vi "Array.vi"() -> ()   [LabVIEW 2018]
panel:
  in  "length":i32
  in  "index":i32
  in  "Mult":dbl
  out "Sub Array":dbl[](array[numeric])
  out "Array final":dbl[](array[numeric])
  out "Array":dbl[](array[numeric])
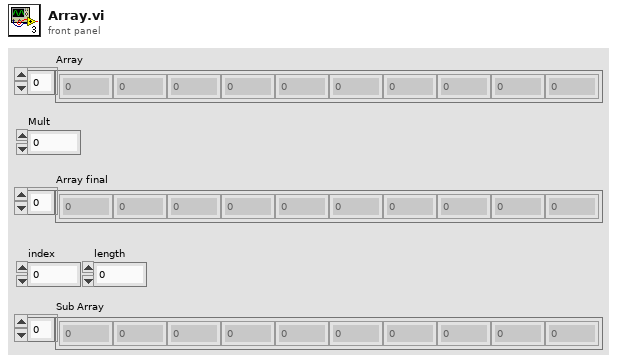
[diagram p1: front panel]
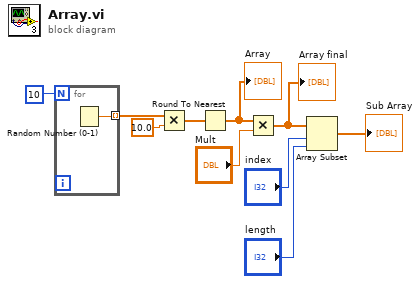
[diagram p0: block diagram]
diagram:
  n1 = for {
    N: 10 -> [_]
    tunnel: [w11] -> w1 mode=indexing
    n2 = Random Number (0-1)() -> (number: 0 to 1=w11:dbl)
  }
  n3 = Multiply(x=w1, y=10.0) -> (x*y=w3:dbl[])
  n4 = Round To Nearest(number=w3) -> (nearest integer value=w2:dbl[])
  "Array" <- w2
  n5 = Multiply(x=w2, y="Mult") -> (x*y=w8:dbl[])
  "Array final" <- w8
  n6 = Array Subset(array=w8, index="index", length="length") -> (→"Sub Array":dbl[])
